vi "Read timing channel offset.vi"(8 "error in (no error)":errorcluster, 11 "Execution Unit in":refnum<class "Execution Unit.lvclass">) -> (0 "error out":errorcluster, 2 "timing channel offset":i64, 3 "Execution Unit out":refnum<class "Execution Unit.lvclass">)   [LabVIEW 2020, in "Ballard ARINC 429 Engine.lvlib" / "Implementation.lvlib" / "Execution Unit.lvclass"]
uses:
  Execution Unit.lvclass
  Execution Unit.lvclass/Execution Unit.ctl
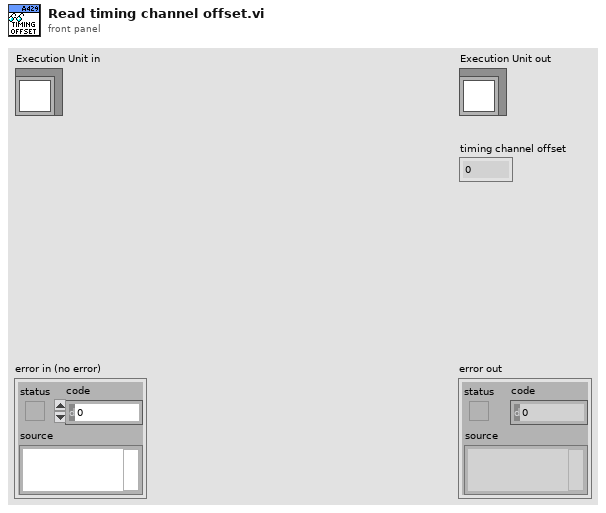
[diagram p1: front panel]
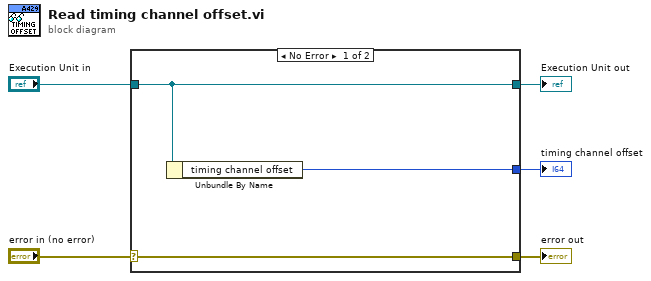
[diagram p0: block diagram]
diagram:
  n1 = case shown="No Error" "error in (no error)" {
    selector: "error in (no error)" -> [w8 w9]
    tunnel: [w8 w9] -> w4
    tunnel: [w7 w10] -> w2
    tunnel: "Execution Unit in" -> [w7 w10]
    tunnel: [w6 _] -> w1
    frame No Error {
      n2 = Unbundle By Name(w7) -> ("timing channel offset"=w6:i64)
    }
    frame Error {
    }
  }
  "error out" <- w4
  "Execution Unit out" <- w2
  "timing channel offset" <- w1
